vi "ThroughPut.vi"() -> ()   [LabVIEW 2014]
uses:
  ClassLibrary1.dll
  <vilib>/Utility/config.llb/NI_LVConfig.lvlib
  MESControldll.dll
panel:
  out "上传MES信息":string
  out "循环检测控制变量":bool=TRUE
  out "测试模式":string
  out "检查批号接受2":string
  out "检查批号接受1":string
  out "barcode":string
  out "MES_mac跳数":string
  out "检查过站信息":string
  out "GZ_NAME":string caption="工站名称"
  out "MES_主键":string
  out "工单号":string
  out "电脑号":string
  out "工站号":string caption="工站名称"
  in  "配置文件键值-Command_info":string[](array[string])=["Client_command", "测试模式"]
  in  "配置文件键值-IP_info":string[](array[string])=["DUT_ip", "Client_ip", "Server_ip"]
  in  "配置文件键值-Param_info":string[](array[string])=["TX标准", "RX标准", "TXRX标准"]
  in  "配置文件键值-MES_info":string[](array[string])=["MES_enable", "MES_主键", "MES_mac跳数", "MES_mac跳数"]
  in  "配置文件键值-GZ_info":string[](array[string])=["工站名称", "工站号", "工号", "电脑号", "工单号"]
  out "工号":string
  out "Client_ip":string
  out "Server_ip":string
  out "Client_command":string
  out "测试信息":string
  out "状态灯":bool
  out "MES指示灯":bool
  out "FAIL数量":string
  out "PASS数量":string
  out "DUT_ip":string
  out "TXRX标准":string
  out "RX标准":string
  out "TX标准":string
  out "MES_enable":string
  out "工站名称":string
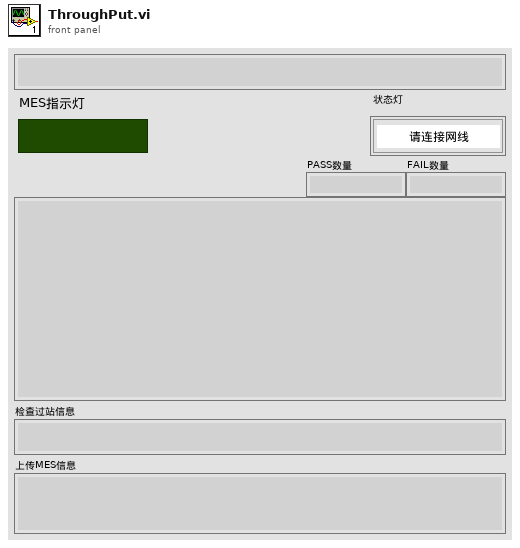
[diagram p1: front panel]
types:
  T1 = typedef "NI_LVConfig.lvlib/Config Data RefNum.ctl" = refnum<k1>
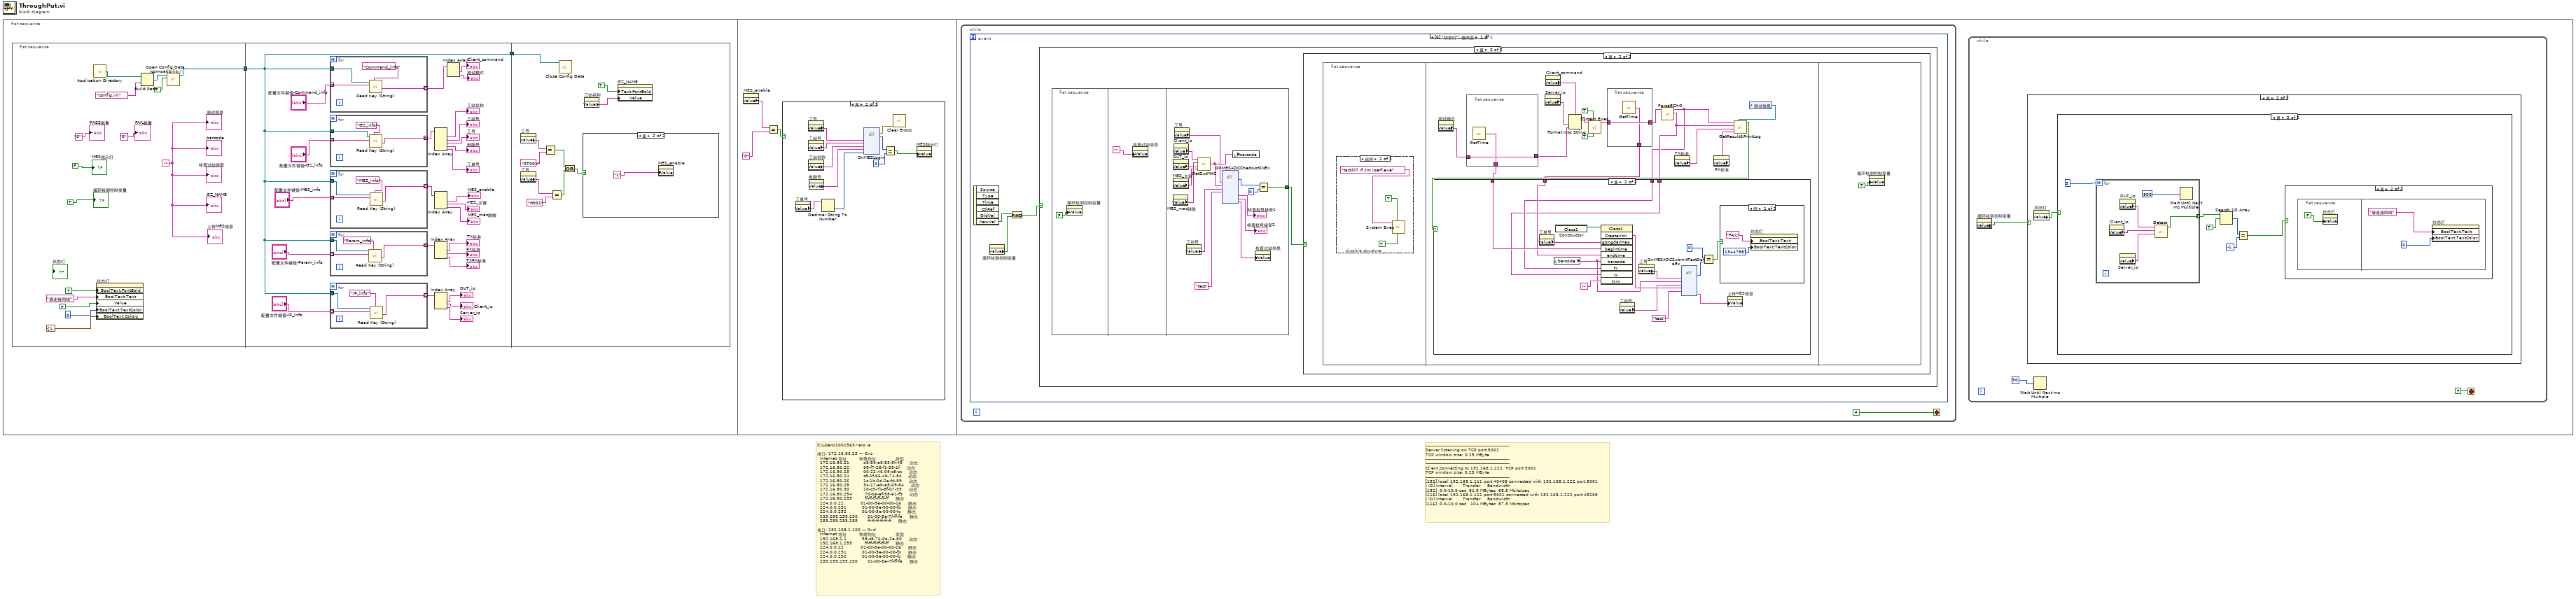
[diagram p0: block diagram]
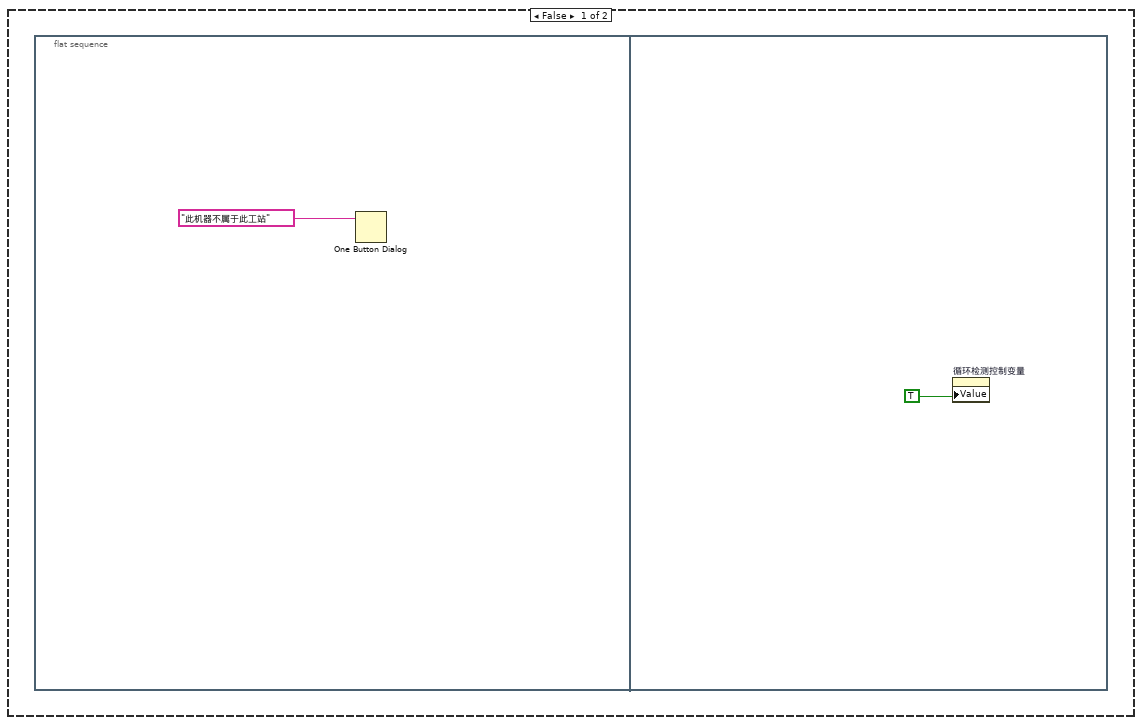
[diagram p5: hidden frame]
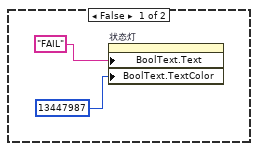
[diagram p7: hidden frame]
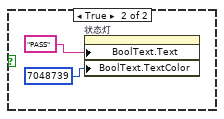
[diagram p8: hidden frame]
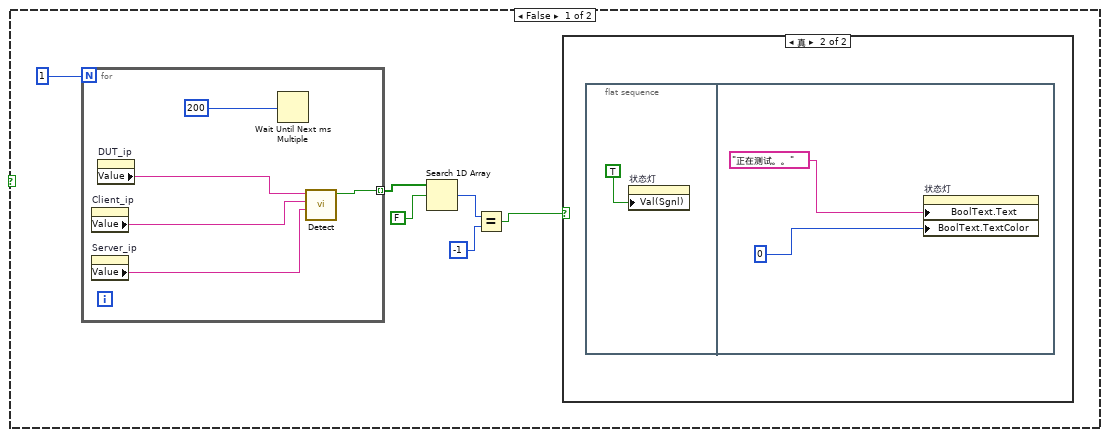
[diagram p10: hidden frame]
diagram:
  # "C:\\Users\\1001563>arp -a\n\n接口: 172.16.80.25 --- 0xc\n  Internet 地址         物理地址              类型\n  172.16.80.21          d8-50-e6-53-5f-45     动态\n  172.16.80.22          68-f7-28-f1-33-1f     动态\n  172.16.80.23          00-22-46-09-c8-cc     动态\n  172.16.80.24          c8-1f-66-4b-74-8c     动态\n  172.16.80.26          1c-1b-0d-2a-fd-89     动态\n  172.16.80.28          34-17-eb-a5-09-84     动态\n  172.16.80.30          10-c3-7b-8f-b7-39     动态\n  172.16.80.254         70-ba-ef-58-a1-f9     动态\n  172.16.80.255         ff-ff-ff-ff-ff-ff     静态\n  224.0.0.22            01-00-5e-00-00-16     静态\n  224.0.0.251           01-00-5e-00-00-fb     静态\n  224.0.0.252           01-00-5e-00-00-fc     静态\n  239.255.255.250       01-00-5e-7f-ff-fa     静态\n  255.255.255.255       ff-ff-ff-ff-ff-ff     静态\n\n接口: 192.168.1.100 --- 0xd\n  Internet 地址         物理地址              类型\n  192.168.1.1           58-c8-76-0a-2a-80     动态\n  192.168.1.255         ff-ff-ff-ff-ff-ff     静态\n  224.0.0.22            01-00-5e-00-00-16     静态\n  224.0.0.251           01-00-5e-00-00-fb     静态\n  224.0.0.252           01-00-5e-00-00-fc     静态\n  239.255.255.250       01-00-5e-7f-ff-fa     静态"
  # "------------------------------------------------------------\nServer listening on TCP port 5001\nTCP window size: 0.25 MByte\n------------------------------------------------------------\n------------------------------------------------------------\nClient connecting to 192.168.1.222, TCP port 5001\nTCP window size: 0.25 MByte\n------------------------------------------------------------\n[152] local 192.168.1.111 port 40408 connected with 192.168.1.222 port 5001\n[ ID] Interval       Transfer     Bandwidth\n[152]  0.0-10.0 sec  81.9 MBytes  68.5 Mbits/sec\n[116] local 192.168.1.111 port 5001 connected with 192.168.1.222 port 49208\n[ ID] Interval       Transfer     Bandwidth\n[116]  0.0-10.0 sec   104 MBytes  87.3 Mbits/sec"
  n1 = flat-sequence {
    frame #0 {
      n2 = flat-sequence {
        tunnel: [w6] -> w1
        tunnel: [w22] -> w2
        tunnel: w1 -> [w22]
        tunnel: w2 -> [w74]
        frame #0 {
          w4 = ""
          n3 = call <vilib>:"Application Directory.vi"() -> ("Application Directory"=w3:path)
          n4 = property on="状态灯" class="Bool (严格)"("BoolText.FontBold"=TRUE, "BoolText.Text"="请连接网线", "Value"=FALSE, "BoolText.TextColor"=0, "BoolText.Colors"=cluster{i32, i32} {16777215, 16777215}) -> ()  [unwired: 2 in, 2 out]
          n5 = Build Path(base path=w3, name or relative path="config.ini") -> (appended path=w11:path)
          n6 = call <vilib>:"Open Config Data (compatibility).vi"("create file if necessary (T)"=FALSE, "configuration file path"=w11) -> ("refnum"=w6:T1)  [unwired: 7 in, 2 out]
          "MES指示灯" <- FALSE
          "PASS数量" <- "0"
          "FAIL数量" <- "0"
          "测试信息" <- w4
          "GZ_NAME" <- w4
          "barcode" <- w4
          "检查过站信息" <- w4
          "循环检测控制变量" <- TRUE
          "上传MES信息" <- w4
        }
        frame #1 {
          n7 = for {
            tunnel: "配置文件键值-Command_info" -> [w64] mode=indexing
            tunnel: w22 -> [w63]
            tunnel: [w61] -> w43 mode=indexing
            n8 = call <vilib>:"Read Key (String).vi"("section"="Command_info", "key"=w64, "refnum"=w63) -> ("value"=w61:string)  [unwired: 5 in, 3 out]
          }
          n9 = for {
            tunnel: "配置文件键值-GZ_info" -> [w59] mode=indexing
            tunnel: w22 -> [w58]
            tunnel: [w57] -> w40 mode=indexing
            n10 = call <vilib>:"Read Key (String).vi"("section"="GZ_info", "key"=w59, "refnum"=w58) -> ("value"=w57:string)  [unwired: 5 in, 3 out]
          }
          n11 = for {
            tunnel: "配置文件键值-MES_info" -> [w55] mode=indexing
            tunnel: w22 -> [w54]
            tunnel: [w53] -> w34 mode=indexing
            n12 = call <vilib>:"Read Key (String).vi"("section"="MES_info", "key"=w55, "refnum"=w54) -> ("value"=w53:string)  [unwired: 5 in, 3 out]
          }
          n13 = for {
            tunnel: "配置文件键值-Param_info" -> [w51] mode=indexing
            tunnel: w22 -> [w50]
            tunnel: [w49] -> w31 mode=indexing
            n14 = call <vilib>:"Read Key (String).vi"("section"="Param_info", "key"=w51, "refnum"=w50) -> ("value"=w49:string)  [unwired: 5 in, 3 out]
          }
          n15 = for {
            tunnel: "配置文件键值-IP_info" -> [w47] mode=indexing
            tunnel: w22 -> [w46]
            tunnel: [w45] -> w26 mode=indexing
            n16 = call <vilib>:"Read Key (String).vi"("section"="IP_info", "key"=w47, "refnum"=w46) -> ("value"=w45:string)  [unwired: 5 in, 3 out]
          }
          n17 = Index Array(array=w40) -> (element #1=→"工站名称":string, element #2=→"工站号":string, element #3=→"工号":string, element #4=→"电脑号":string, element #5=→"工单号":string)  [unwired: 5 in]
          n18 = Index Array(array=w34) -> (element #1=→"MES_enable":string, element #2=→"MES_主键":string, element #3=→"MES_mac跳数":string)  [unwired: 3 in]
          n19 = Index Array(array=w31) -> (element #1=→"TX标准":string, element #2=→"RX标准":string, element #3=→"TXRX标准":string)  [unwired: 3 in]
          n20 = Index Array(array=w26) -> (element #1=→"DUT_ip":string, element #2=→"Client_ip":string, element #3=→"Server_ip":string)  [unwired: 3 in]
          n21 = Index Array(array=w43) -> (element #1=→"Client_command":string, element #2=→"测试模式":string)  [unwired: 2 in]
        }
        frame #2 {
          n22 = property on="工号" class="Str"() -> ("Value"=w70:string)  [unwired: 2 in, 2 out]
          n23 = property on="工号" class="Str"() -> ("Value"=w73:string)  [unwired: 2 in, 2 out]
          n24 = Equal?(x=w70, y="RT001") -> (x = y?=w69:bool)
          n25 = Equal?(x=w73, y="rt001") -> (x = y?=w68:bool)
          n26 = call <vilib>:"Close Config Data.vi"("refnum"=w74) -> ()  [unwired: 9 in, 2 out]
          n27 = Or(x=w69, y=w68) -> (x .or. y?=w67:bool)
          n28 = case shown="真" w67 {
            frame False {
            }
            frame True {
              n29 = property on="MES_enable" class="Str"("Value"="1") -> ()  [unwired: 2 in, 2 out]
            }
          }
          n30 = property on="工站名称" class="Str"() -> ("Value"=w65:string)  [unwired: 2 in, 2 out]
          n31 = property on="GZ_NAME" class="Str"("Text.FontBold"=TRUE, "Value"=w65) -> ()  [unwired: 2 in, 2 out]
        }
      }
    }
    frame #1 {
      n32 = property on="MES_enable" class="Str"() -> ("Value"=w78:string)  [unwired: 2 in, 2 out]
      n33 = Equal?(x=w78, y="0") -> (x = y?=w76:bool)
      n34 = case shown="真" w76 {
        frame False {
        }
        frame True {
          n35 = property on="工单号" class="Str"() -> ("Value"=w84:string)  [unwired: 2 in, 2 out]
          n36 = property on="工号" class="Str"() -> ("Value"=w88:string)  [unwired: 2 in, 2 out]
          n37 = property on="工站号" class="Str"() -> ("Value"=w87:string)  [unwired: 2 in, 2 out]
          n38 = property on="工站名称" class="Str"() -> ("Value"=w86:string)  [unwired: 2 in, 2 out]
          n39 = property on="电脑号" class="Str"() -> ("Value"=w85:string)  [unwired: 2 in, 2 out]
          n40 = Decimal String To Number(string=w84) -> (number=w83:i32)  [unwired: 2 in, 1 out]
          n41 = dll-call lib="PTH2Dabs CUsers1001563Desktop自写吞吐量MESControldll.dll" fn="OnMESLogin"("userid"=w88, "PointNum"=w87, "PointName"=w86, "PCname"=w85, "GongDanNum"=w83) -> (error out=w79:errorcluster, "result"=w81:i32)  [unwired: 8 in, 1 out]
          n42 = Equal?(x=w81, y=0) -> (x = y?=w80:bool)
          n43 = call <vilib>:"Clear Errors.vi"("error in (no error)"=w79) -> ()  [unwired: 5 in, 2 out]
          n44 = property on="MES指示灯" class="Bool (严格)"("Value"=w80) -> ()  [unwired: 2 in, 2 out]
        }
      }
    }
    frame #2 {
      n45 = while {
        stop <- FALSE stop-if-true
        n46 = event shown="[0] \"状态灯\": 值改变" {
          selector: _ -> [_]
          dyn-events: _ -> [_]
          timeout: _ -> [_]
          event "状态灯": Value Change {
            n47 = event-data() -> ("NewVal"=w91:bool)  [unwired: 1 in, 5 out]
            n48 = property on="循环检测控制变量" class="Bool (严格)"() -> ("Value"=w92:bool)  [unwired: 2 in, 2 out]
            n49 = And(x=w91, y=w92) -> (x .and. y?=w90:bool)
            n50 = case shown="真" w90 {
              frame False {
              }
              frame True {
                n51 = flat-sequence {
                  tunnel: [w104] -> w93
                  frame #0 {
                    n52 = property on="循环检测控制变量" class="Bool (严格)"("Value"=FALSE) -> ()  [unwired: 2 in, 2 out]
                  }
                  frame #1 {
                    n53 = property on="检查过站信息" class="Str"("Value"="") -> ()  [unwired: 2 in, 2 out]
                  }
                  frame #2 {
                    n54 = property on="MES_mac跳数" class="Str"() -> ("Value"=w103:string)  [unwired: 2 in, 2 out]
                    n55 = property on="DUT_ip" class="Str"() -> ("Value"=w101:string)  [unwired: 2 in, 2 out]
                    n56 = property on="MES_主键" class="Str"() -> ("Value"=w102:string)  [unwired: 2 in, 2 out]
                    n57 = property on="Client_ip" class="Str"() -> ("Value"=w100:string)  [unwired: 2 in, 2 out]
                    n58 = property on="工号" class="Str"() -> ("Value"=w109:string)  [unwired: 2 in, 2 out]
                    n59 = property on="工站号" class="Str"() -> ("Value"=w108:string)  [unwired: 2 in, 2 out]
                    n60 = call "GetDutMAC.vi"("MAC模式"=w102, "Dut_ip"=w101, "MAC跳数"=w103, "Client_ip"=w100) -> ("输出MAC"=w99:string)
                    n61 = dll-call lib="PTH2Dabs CUsers1001563Desktop自写吞吐量MESControldll.dll" fn="OnMESADCCheckLotSNEx"("userid"=w109, "barcode"=w99, "PointNum"=w108, "SheetName"="test") -> ("result"=w106:i32, "ReKong"=→"检查批号接受1":string, "ReGongDanNum"=→"检查批号接受2":string, "ReInfo"=w96:string)  [unwired: 10 in, 2 out]
                    n62 = local write "barcode"(w99) -> ()
                    n63 = property on="检查过站信息" class="Str"("Value"=w96) -> ()  [unwired: 2 in, 2 out]
                    n64 = Equal?(x=w106, y=0) -> (x = y?=w104:bool)
                  }
                }
                n65 = case shown="真" w93 {
                  frame False {
                    n66 = flat-sequence {
                      frame #0 {
                        n67 = One Button Dialog(message="此机器不属于此工站") -> ()  [unwired: 1 in, 1 out]
                      }
                      frame #1 {
                        n68 = property on="循环检测控制变量" class="Bool (严格)"("Value"=TRUE) -> ()  [unwired: 2 in, 2 out]
                      }
                    }
                  }
                  frame True {
                    n69 = flat-sequence {
                      frame #0 {
                        n70 = disable-structure shown="启用" {
                          frame Disabled {
                          }
                          frame Enabled {
                            n71 = call <vilib>:"System Exec.vi"("run minimized? (F)"=TRUE, "wait until completion? (T)"=TRUE, "command line"="taskkill /f /im iperf.exe") -> ()  [unwired: 5 in, 4 out]
                          }
                        }
                      }
                      frame #1 {
                        n72 = property on="测试模式" class="Str"() -> ("Value"=w122:string)  [unwired: 2 in, 2 out]
                        n73 = flat-sequence {
                          tunnel: w122 -> [w135]
                          tunnel: [w135] -> w121
                          tunnel: [w134] -> w120
                          frame #0 {
                            n74 = call "GetTime.vi"() -> ("输出"=w134:string)  [unwired: 1 in]
                          }
                        }
                        n75 = property on="Server_ip" class="Str"() -> ("Value"=w130:string)  [unwired: 2 in, 2 out]
                        n76 = property on="Client_command" class="Str"() -> ("Value"=w131:string)  [unwired: 2 in, 2 out]
                        n77 = Format Into String(format string=w131, w130, w121) -> (resulting string=w129:string)  [unwired: 2 in, 1 out]
                        n78 = call <vilib>:"System Exec.vi"("run minimized? (F)"=TRUE, "wait until completion? (T)"=TRUE, "command line"=w129) -> ("standard output"=w119:string)  [unwired: 5 in, 3 out]
                        n79 = flat-sequence {
                          tunnel: [w133] -> w118
                          tunnel: w119 -> [w133]
                          tunnel: [w132] -> w117
                          frame #0 {
                            n80 = call "GetTime.vi"() -> ("输出"=w132:string)  [unwired: 1 in]
                          }
                        }
                        n81 = call "ParseECHO.vi"("指令返回的字符串"=w118) -> ("RX测量"=w116:string, "TX测量"=w115:string)  [unwired: 7 in]
                        n82 = property on="TX标准" class="Str"() -> ("Value"=w125:string)  [unwired: 2 in, 2 out]
                        n83 = property on="RX标准" class="Str"() -> ("Value"=w124:string)  [unwired: 2 in, 2 out]
                        n84 = control-ref of="测试信息"() -> (w126:refnum<vi>)
                        n85 = call "GetResult&PrintLog.vi"("Str引用句柄"=w126, "RX标准"=w124, "TX标准"=w125, "RX测量"=w116, "TX测量"=w115) -> ("布尔"=w123:bool)  [unwired: 4 in]
                        n86 = case shown="真" w123 {
                          tunnel: w120 -> [_ w151]
                          tunnel: w117 -> [_ w150]
                          tunnel: w115 -> [_ w149]
                          tunnel: w116 -> [_ w148]
                          frame False {
                            n87 = property on="状态灯" class="Bool (严格)"("BoolText.Text"="FAIL", "BoolText.TextColor"=13447987) -> ()  [unwired: 2 in, 2 out]
                          }
                          frame True {
                            n88 = property on="工单号" class="Str"() -> ("Value"=w152:string)  [unwired: 2 in, 2 out]
                            n89 = local read "barcode"() -> (w146:string)
                            n90 = constructor class="Class1"() -> (reference out=w153:refnum<k24>)  [unwired: 3 in, 2 out]
                            n91 = invoke on="调用节点" class="Class1" method="CreateXml"(reference=w153, "gongdanhao"=w152, "begintime"=w151, "endtime"=w150, "barcode"=w146, "tx"=w149, "rx"=w148, "txrx"="") -> ("CreateXml"=w143:string)  [unwired: 2 in, 9 out]
                            n92 = property on="工站号" class="Str"() -> ("Value"=w144:string)  [unwired: 2 in, 2 out]
                            n93 = property on="工号" class="Str"() -> ("Value"=w145:string)  [unwired: 2 in, 2 out]
                            n94 = dll-call lib="PTH2Dabs CUsers1001563Desktop自写吞吐量MESControldll.dll" fn="OnMESADCSubmitTestDataEx"("userid"=w145, "barcode"=w146, "pointName"=w144, "ParamVal"=w143, "postcode"="test") -> ("result"=w139:i32, "errbuf"=w141:string)  [unwired: 9 in, 2 out]
                            n95 = Equal?(x=0, y=w139) -> (x = y?=w138:bool)
                            n96 = case shown="假" w138 {
                              frame False {
                                n97 = property on="状态灯" class="Bool (严格)"("BoolText.Text"="FAIL", "BoolText.TextColor"=13447987) -> ()  [unwired: 2 in, 2 out]
                              }
                              frame True {
                                n98 = property on="状态灯" class="Bool (严格)"("BoolText.Text"="PASS", "BoolText.TextColor"=7048739) -> ()  [unwired: 2 in, 2 out]
                              }
                            }
                            n99 = property on="上传MES信息" class="Str"("Value"=w141) -> ()  [unwired: 2 in, 2 out]
                          }
                        }
                      }
                      frame #2 {
                        n100 = property on="循环检测控制变量" class="Bool (严格)"("Value"=TRUE) -> ()  [unwired: 2 in, 2 out]
                      }
                    }
                  }
                }
              }
            }
          }
        }
      }
      n101 = while {
        stop <- FALSE stop-if-true
        n102 = property on="循环检测控制变量" class="Bool (严格)"() -> ("Value"=w159:bool)  [unwired: 2 in, 2 out]
        n103 = case shown="真" w159 {
          frame False {
          }
          frame True {
            n104 = property on="状态灯" class="Bool (严格)"() -> ("Value"=w162:bool)  [unwired: 2 in, 2 out]
            n105 = case shown="真" w162 {
              frame False {
                n106 = for {
                  N: 1 -> [_]
                  tunnel: [w173] -> w167 mode=indexing
                  n107 = property on="Client_ip" class="Str"() -> ("Value"=w175:string)  [unwired: 2 in, 2 out]
                  n108 = property on="Server_ip" class="Str"() -> ("Value"=w174:string)  [unwired: 2 in, 2 out]
                  n109 = property on="DUT_ip" class="Str"() -> ("Value"=w176:string)  [unwired: 2 in, 2 out]
                  n110 = Wait Until Next ms Multiple(millisecond multiple=200) -> ()  [unwired: 1 out]
                  n111 = call "Detect.vi"("server-ip"=w174, "client-ip"=w175, "dut-ip"=w176) -> ("布尔"=w173:bool)  [unwired: 3 in, 1 out]
                }
                n112 = Search 1D Array(1D array=w167, element=FALSE) -> (index of element=w164:i32)  [unwired: 1 in]
                n113 = Equal?(x=w164, y=-1) -> (x = y?=w163:bool)
                n114 = case shown="真" w163 {
                  frame False {
                  }
                  frame True {
                    n115 = flat-sequence {
                      frame #0 {
                        n116 = property on="状态灯" class="Bool (严格)"("Val(Sgnl)"=TRUE) -> ()  [unwired: 2 in, 2 out]
                      }
                      frame #1 {
                        n117 = property on="状态灯" class="Bool (严格)"("BoolText.Text"="正在测试。。", "BoolText.TextColor"=0) -> ()  [unwired: 2 in, 2 out]
                      }
                    }
                  }
                }
              }
              frame True {
                n118 = for {
                  N: 3 -> [_]
                  tunnel: [w183] -> w181 mode=indexing
                  n119 = property on="Client_ip" class="Str"() -> ("Value"=w185:string)  [unwired: 2 in, 2 out]
                  n120 = property on="DUT_ip" class="Str"() -> ("Value"=w187:string)  [unwired: 2 in, 2 out]
                  n121 = property on="Server_ip" class="Str"() -> ("Value"=w186:string)  [unwired: 2 in, 2 out]
                  n122 = call "Detect.vi"("server-ip"=w186, "client-ip"=w185, "dut-ip"=w187) -> ("布尔"=w183:bool)  [unwired: 3 in, 1 out]
                  n123 = Wait Until Next ms Multiple(millisecond multiple=800) -> ()  [unwired: 1 out]
                }
                n124 = Search 1D Array(1D array=w181, element=TRUE) -> (index of element=w178:i32)  [unwired: 1 in]
                n125 = Equal?(x=w178, y=-1) -> (x = y?=w177:bool)
                n126 = case shown="真" w177 {
                  frame False {
                  }
                  frame True {
                    n127 = flat-sequence {
                      frame #0 {
                        n128 = property on="状态灯" class="Bool (严格)"("Value"=FALSE) -> ()  [unwired: 2 in, 2 out]
                      }
                      frame #1 {
                        n129 = property on="状态灯" class="Bool (严格)"("BoolText.Text"="请连接网线", "BoolText.TextColor"=0) -> ()  [unwired: 2 in, 2 out]
                      }
                    }
                  }
                }
              }
            }
          }
        }
        n130 = Wait Until Next ms Multiple(millisecond multiple=50) -> ()  [unwired: 1 out]
      }
    }
  }
